vi "CRYFlatten Test Infor.vi"(11 "Test Infor data":T1) -> (3 "Fattened Data":string)   [LabVIEW 2013]
uses:
  Typedef Control/CRYStimulus Test Infor Cluster.ctl
panel:
  out "FreqAmpPhase":cluster{"freq":dbl, "ampl":dbl, "cycles":dbl}[](array[cluster]) {"cycles" format="%.2f"; "ampl" format="%.2f"; "freq" format="%.2f"}
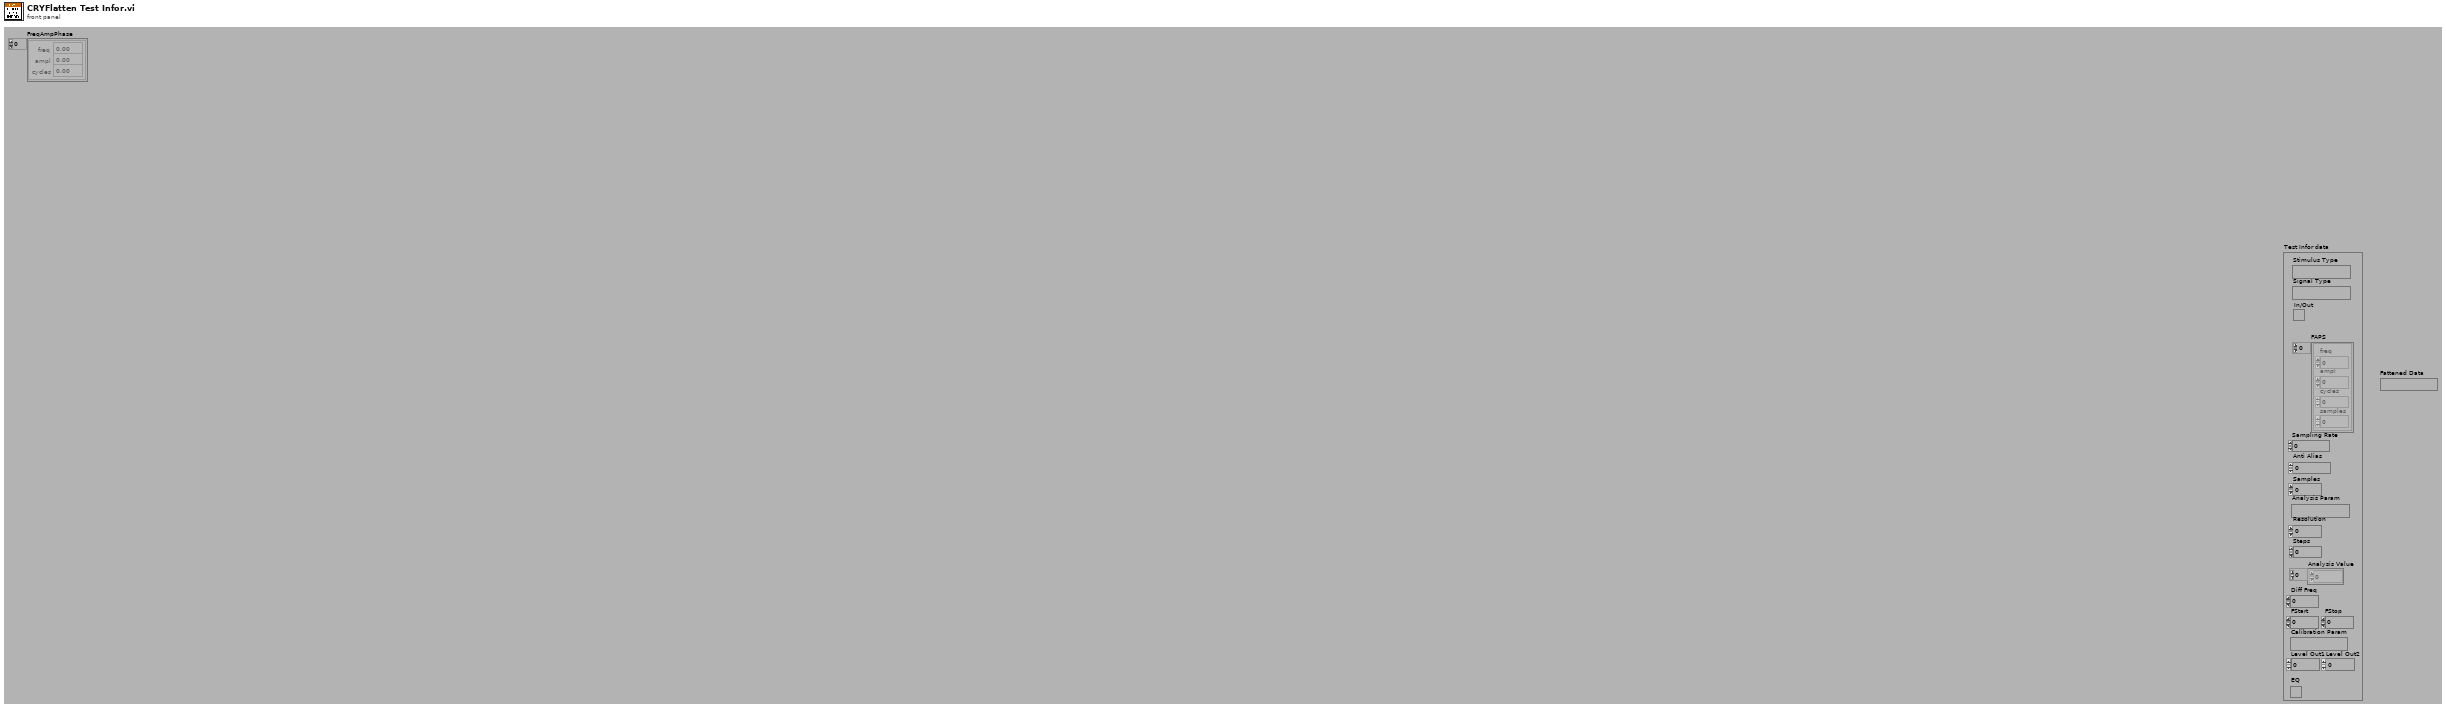
[diagram p1: front panel]
types:
  T1 = typedef "CRYStimulus Test Infor Cluster.ctl" = cluster{"Stimulus Type":string, "Signal Type":string, "In/Out":bool, "FAPS":cluster{"freq":dbl, "ampl":dbl, "cycles":dbl, "samples":i32}[], "Sampling Rate":dbl, "Samples":i32, "Analysis Param":string, "Resolution":u16, "Steps":u32, "Analysis Value":dbl[], "Diff Freq":dbl, "FStart":dbl, "FStop":dbl, "Calibration Param":string, "Anti Alias":dbl, "Level Out1":dbl, "Level Out2":dbl, "EQ":bool}
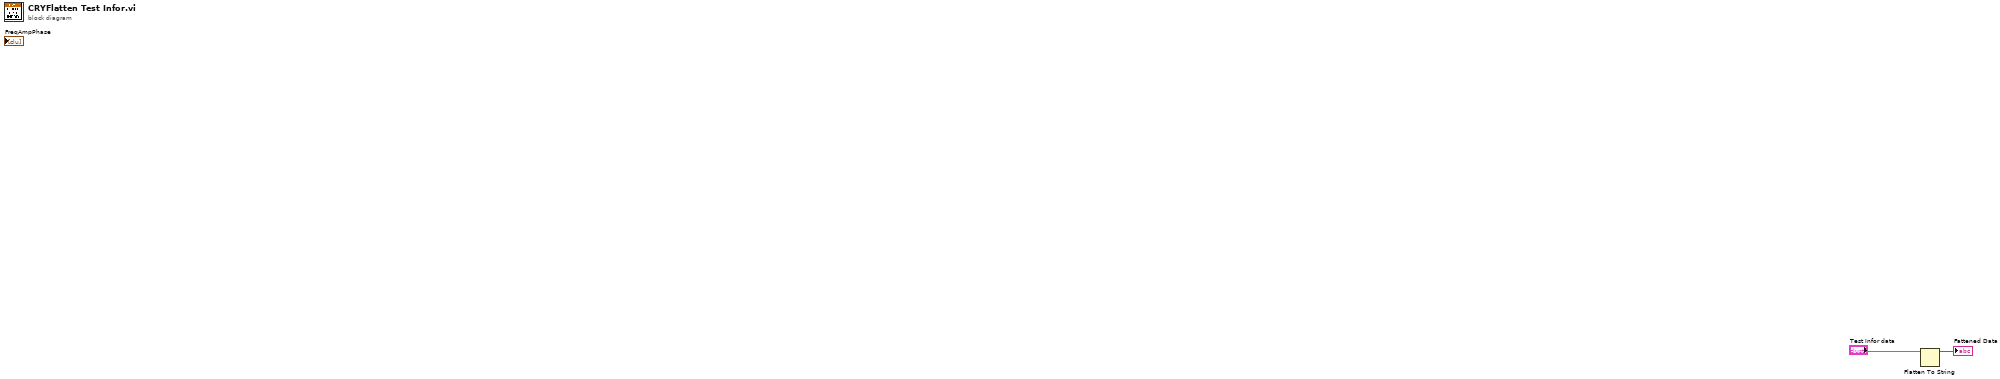
[diagram p0: block diagram]
diagram:
  n1 = Flatten To String(anything="Test Infor data") -> (data string=→"Fattened Data":string)  [unwired: 1 in, 4 out]
